vi "Get if Loop Sequence.vi"(8 "error in (no error)":errorcluster caption="entrée d'erreur (pas d'erreur)", 10 "Function":T1(ring), 11 "Loop In":bool) -> (0 "error out":errorcluster caption="sortie d'erreur", 3 "Loop Out":bool)   [LabVIEW 2020]
uses:
  TypeDef/Variable Printable.ctl
  Library Commun.lvlib
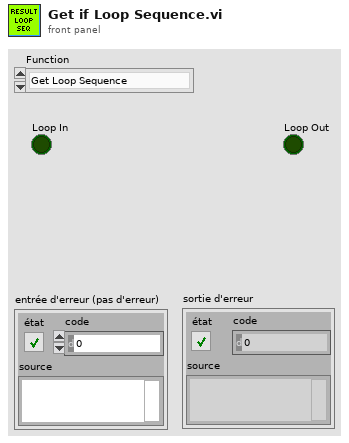
[diagram p1: front panel]
types:
  T1 = enum16{"Get Loop Sequence", "Reset", "Set Loop Sequence"}
  T2 = typedef "Variable Printable.ctl" = string
  T3 = enum16{"Get Variable", "Get All Variables", "Set Variable", "Delete Variable", "Delete All Variable"}
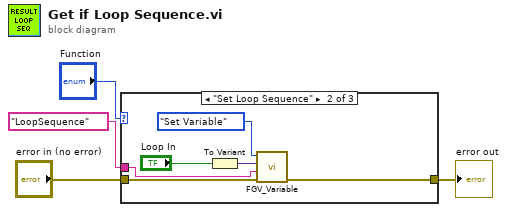
[diagram p0: block diagram]
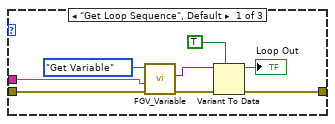
[diagram p2: hidden frame]
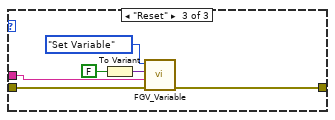
[diagram p3: hidden frame]
diagram:
  n1 = case shown="\"Set Loop Sequence\"" "Function" {
    tunnel: T2 "LoopSequence" ("Variable") -> [w11 w13 w24]
    tunnel: "error in (no error)" -> [w10 w14 w19]
    tunnel: [w8 w18 w23] -> w2
    frame "Get Loop Sequence", Default {
      n2 = call "FGV_Variable.vi"("error in (no error)"=w10, "Variable"=w11, "Function"=T3."Get Variable") -> ("error out"=w9:errorcluster, "Data Out"=w7:variant)  [unwired: 6 in, 1 out]
      n3 = Variant To Data(error in=w9, type=TRUE, Variant=w7) -> (data=→"Loop Out":bool, error out=w8:errorcluster)
    }
    frame "Set Loop Sequence" {
      n4 = To Variant(anything="Loop In") -> (Variant=w15:variant)
      n5 = call "FGV_Variable.vi"("error in (no error)"=w14, "Variable"=w13, "Data In"=w15, "Function"=T3."Set Variable") -> ("error out"=w18:errorcluster)  [unwired: 5 in, 2 out]
    }
    frame "Reset" {
      n6 = To Variant(anything=FALSE) -> (Variant=w21:variant)
      n7 = call "FGV_Variable.vi"("error in (no error)"=w19, "Variable"=w24, "Data In"=w21, "Function"=T3."Set Variable") -> ("error out"=w23:errorcluster)  [unwired: 5 in, 2 out]
    }
  }
  "error out" <- w2
